vi "Search 1D String Array by Pattern.vi"(4 "Reg text":string, 5 "1D String Array":string[](array[string])) -> (1 "index of element":i32)   [LabVIEW 2017, in "API String Arguments Support.lvlib"]
uses:
  API String Arguments Support.lvlib
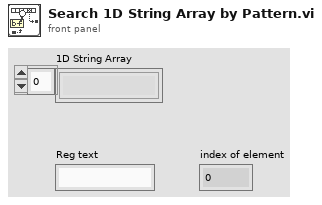
[diagram p1: front panel]
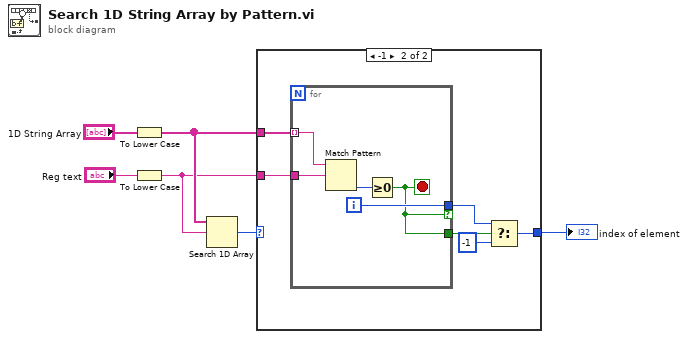
[diagram p0: block diagram]
diagram:
  n1 = To Lower Case(string="1D String Array") -> (all lower case string=w3:string[])
  n2 = To Lower Case(string="Reg text") -> (all lower case string=w2:string)
  n3 = Search 1D Array(1D array=w3, element=w2) -> (index of element=w1:i32)  [unwired: 1 in]
  n4 = case shown="-1" w1 {
    selector: w1 -> [w7 _]
    tunnel: [w7 w13] -> w6
    tunnel: w3 -> [_ w9]
    tunnel: w2 -> [_ w8]
    frame Default {
    }
    frame -1 {
      n5 = for {
        tunnel: w9 -> [w18] mode=indexing
        tunnel: w8 -> [w17]
        tunnel: [w16] -> w11 if=w14
        tunnel: [w14] -> w10
        i -> [w16]
        stop <- w14 stop-if-true
        n6 = Match Pattern(string=w18, regular expression=w17) -> (offset past match=w15:i32)  [unwired: 1 in, 3 out]
        n7 = Greater Or Equal To 0?(x=w15) -> (x >= 0?=w14:bool)
      }
      n8 = Select(t=w11, s=w10, f=-1) -> (s? t:f=w13:i32)
    }
  }
  "index of element" <- w6
